vi "Read ErrorColorText.vi"(8 "error in (no error)":errorcluster, 11 "PhoneFromField in":refnum<class "PhoneFromField.lvclass">) -> (0 "error out":errorcluster, 2 "CorrectColorBG":u32(colorbox), 3 "PhoneFromField out":refnum<class "PhoneFromField.lvclass">)   [LabVIEW 2019, in "PhoneFromField.lvclass"]
uses:
  PhoneFromField.lvclass
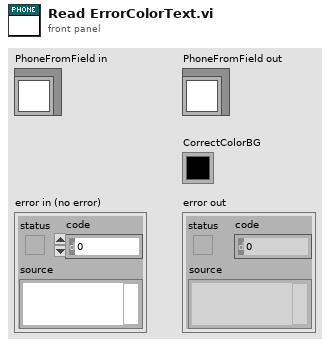
[diagram p1: front panel]
types:
  T1 = typedef "PhoneFromField.lvclass/State Data.ctl" = cluster{"CorrectColorBG":u32}
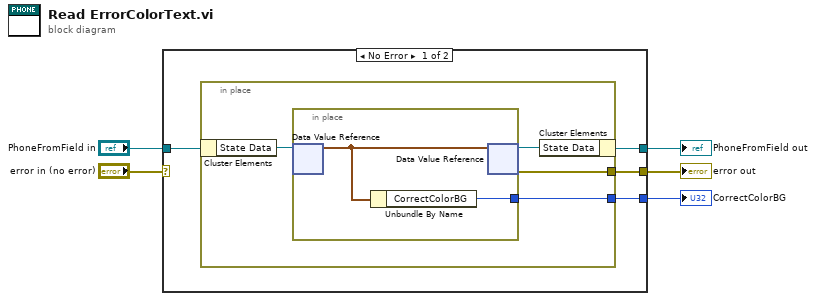
[diagram p0: block diagram]
diagram:
  n1 = case shown="No Error" "error in (no error)" {
    selector: "error in (no error)" -> [_ w17]
    tunnel: [w7 w17] -> w4
    tunnel: [w8 w16] -> w2
    tunnel: "PhoneFromField in" -> [w9 w16]
    tunnel: [w6 _] -> w1
    frame No Error {
      n2 = in-place {
        in-place-border: [w11] -> w7
        in-place-border: [w10] -> w6
        n3 = in-place-cluster #1(w9) -> ("State Data"=w13:refnum<data-value>)
        n4 = in-place {
          in-place-border: [w14] -> w10
          n5 = in-place-dvr #2(w13) -> (w15:T1)  [unwired: 1 out]
          n6 = Unbundle By Name(w15) -> ("CorrectColorBG"=w14:u32)
          n7 = in-place-dvr #2(w15) -> (w12:refnum<data-value>, w11:errorcluster)
        }
        n8 = in-place-cluster #1("State Data"=w12) -> (w8:refnum<class "PhoneFromField.lvclass">)
      }
    }
    frame Error {
    }
  }
  "error out" <- w4
  "PhoneFromField out" <- w2
  "CorrectColorBG" <- w1
